vi "Global 1.vi"() -> ()   [LabVIEW 2016]
panel:
  out "Checkpoint 1":bool
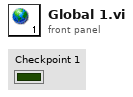
[diagram p1: front panel]
diagram:
